vi "getCompressionParams.vi"(0 "Camera in":refnum<class "Camera.lvclass">, 11 "error in (no error)":errorcluster) -> (4 "Camera out":refnum<class "Camera.lvclass">, 6 "PCO_Recorder_CompressionParams":T1, 15 "error out":errorcluster)   [LabVIEW 2019, in "Camera.lvclass"]
doc: "Retreive the rec handle.\nThis handle allows direct access to all underlying functions of the pco.recorder."
uses:
  Camera.lvclass
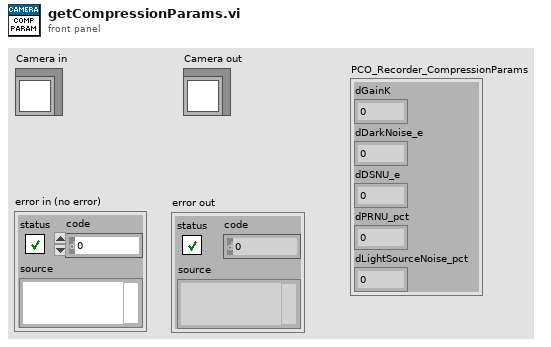
[diagram p1: front panel]
types:
  T1 = cluster{"dGainK":dbl, "dDarkNoise_e":dbl, "dDSNU_e":dbl, "dPRNU_pct":dbl, "dLightSourceNoise_pct":dbl}
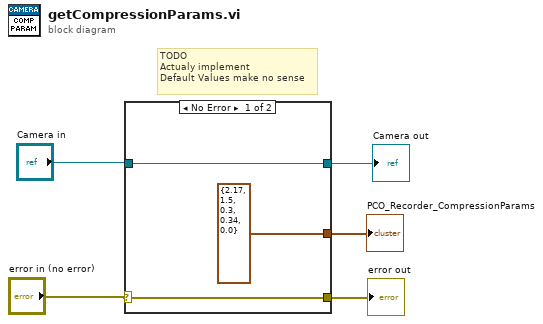
[diagram p0: block diagram]
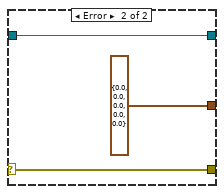
[diagram p2: hidden frame]
diagram:
  # "TODO\nActualy implement\nDefault Values make no sense"
  n1 = case shown="No Error" "error in (no error)" {
    selector: "error in (no error)" -> [w7 w11]
    tunnel: [w7 w11] -> w3
    tunnel: [w8 w10] -> w4
    tunnel: "Camera in" -> [w8 w10]
    tunnel: [T1 {"dGainK"=2.17, "dDarkNoise_e"=1.5, "dDSNU_e"=0.3, "dPRNU_pct"=0.34, "dLightSourceNoise_pct"=0.0} ("PCO_Recorder_CompressionParams") T1 {"dGainK"=0.0, "dDarkNoise_e"=0.0, "dDSNU_e"=0.0, "dPRNU_pct"=0.0, "dLightSourceNoise_pct"=0.0} ("PCO_Recorder_CompressionParams")] -> w1
    frame No Error {
    }
    frame Error {
    }
  }
  "error out" <- w3
  "Camera out" <- w4
  "PCO_Recorder_CompressionParams" <- w1
